vi "TEST_JPEG.vi"() -> ()   [LabVIEW 2009]
uses:
  <vilib>/picture/picture.llb/imagedata.ctl
  SRV VIs/ImageProcessing/QT_Image.ctl
panel:
  out "error out 2":errorcluster
  out "length":i32
  out "data":string
  out "size of data":i32
  out "dimensions":cluster{"Witdh":i32, "Height":i32}
  out "image":picture
  out "Image/Movie Out":T1 {"Dialogs" format="%.0b"}
  out "error out":errorcluster
  out "image data":T2
  in  "path to JPEG file":path=path "C:/Users/Michael.Schultz/AppData/Local/Temp/temp.jpg"
  # "6.17 KB (6,321 bytes)"
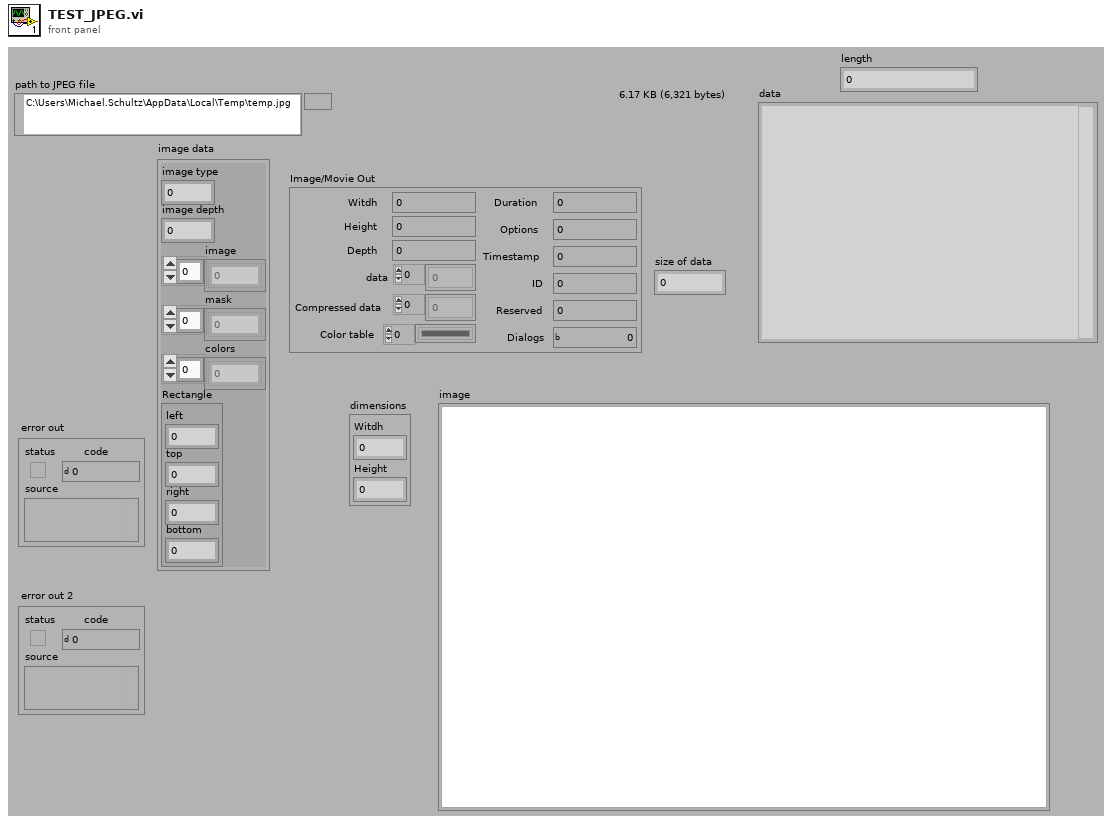
[diagram p1: front panel]
types:
  T1 = typedef "QT_Image.ctl" = cluster{"Witdh":i32, "Height":i32, "Depth":i32, "data":u8[], "Compressed data":u8[], "Color table":u32[], "Duration":i32, "Options":i32, "Timestamp":i32, "ID":i32, "Reserved":i32, "Dialogs":u32}
  T2 = typedef "imagedata.ctl" = cluster{"image type":i32, "image depth":i32, "image":u8[], "mask":u8[], "colors":u32[], "Rectangle":cluster{"left":i16, "top":i16, "right":i16, "bottom":i16}}
  T3 = enum16{"big-endian, network order", "native, host order", "little-endian"}
  T4 = enum16{"No Change", "Apricot", "Carnation", "Ether", "Greyscale", "Greyscale-banded", "Hot Metal", "Lava Waves", "Mac", "Morning Glory", "Rainbow", "Rainbow-banded", "Rainbow-inverted", "Rainbow-striped", "Saturn", "Seismic", "Space"}
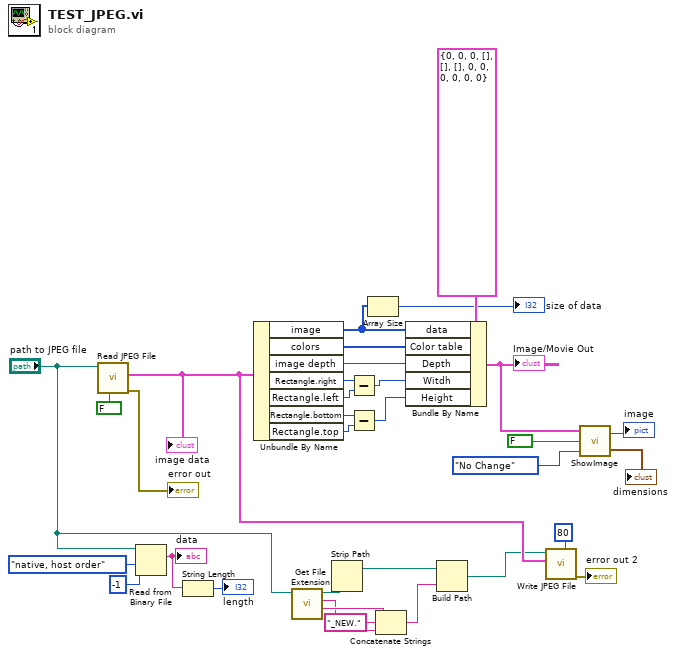
[diagram p0: block diagram]
diagram:
  n1 = call <vilib>:"Read JPEG File.vi"("use 8 bit color table"=FALSE, "path to JPEG file"="path to JPEG file") -> ("error out"=→"error out":errorcluster, "image data"=w11:T2)  [unwired: 7 in, 1 out]
  "image data" <- w11
  n2 = Read from Binary File(9:T3."native, host order" ("byte order (0:big-endian, network order)"), 10:-1 ("count (1)"), 11:"path to JPEG file") -> (2:w14:string)  [unwired: 3 in, 3 out]
  "data" <- w14
  n3 = String Length(string=w14) -> (length=→"length":i32)
  n4 = Unbundle By Name(w11) -> ("image"=w18:u8[], "colors"=w23:u32[], "image depth"=w24:i32, "Rectangle.right"=w25:i16, "Rectangle.left"=w26:i16, "Rectangle.bottom"=w29:i16, "Rectangle.top"=w30:i16)
  n5 = call <vilib>:"Get File Extension.vi"("file"="path to JPEG file") -> ("filename without extension"=w6:string, "lowercase file extension"=w4:string, "dup file"=w7:path)  [unwired: 7 in, 1 out]
  n6 = Strip Path(path=w7) -> (stripped path=w9:path)  [unwired: 1 out]
  n7 = Subtract(x=w25, y=w26) -> (x-y=w27:i16)
  n8 = Subtract(x=w29, y=w30) -> (x-y=w28:i16)
  n9 = Array Size(array=w18) -> (size(s)=→"size of data":i32)
  n10 = Concatenate Strings(w6, "_NEW." ("string"), w4) -> (w3:string)
  n11 = Bundle By Name(cluster=T1 {"Witdh"=0, "Height"=0, "Depth"=0, "data"=[], "Compressed data"=[], "Color table"=[], "Duration"=0, "Options"=0, "Timestamp"=0, "ID"=0, "Reserved"=0, "Dialogs"=0} ("Image Setting"), "data"=w18, "Color table"=w23, "Depth"=w24, "Witdh"=w27, "Height"=w28) -> (w12:T1)
  "Image/Movie Out" <- w12
  n12 = Build Path(base path=w9, name or relative path=w3) -> (appended path=w2:path)
  n13 = call <vilib>:"Write JPEG File.vi"("quality (80)"=80, "image data"=w11, "path to JPEG file"=w2) -> ("error out"=→"error out 2":errorcluster)  [unwired: 7 in, 1 out]
  n14 = call "ShowImage.vi"("Color Table"=T4."No Change", "Autoscale?"=FALSE ("Autoscale? (F)"), "Image"=w12) -> ("dimensions"=→"dimensions":cluster{"Witdh":i32, "Height":i32}, "image"=→"image":picture)
